vi "get_stage_info.vi"(8 "error in (no error)":errorcluster, 10 "repo_type":string, 11 "node in":refnum<k20>) -> (0 "error out":errorcluster, 2 "Stage info":T1(array[cluster]), 3 "node out":refnum<k20>)   [LabVIEW 2010, in "XML_repo_library.lvlib"]
uses:
  XML_repo_library.lvlib
  <vilib>/xml/Close Reference(Node).vi
  <vilib>/xml/NI_XML.lvlib
  C:/Program Files (x86)/National Instruments/LabVIEW 2010/resource/objmgr/DOMUserDefRef.rc
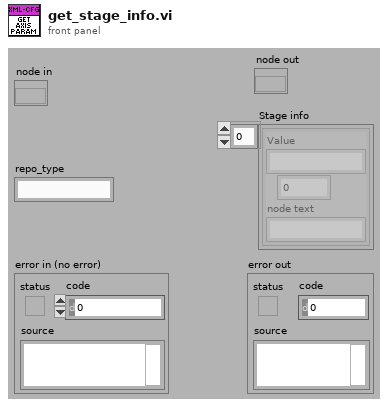
[diagram p1: front panel]
types:
  T1 = cluster{"Value":string, i32, "node text":string}[]
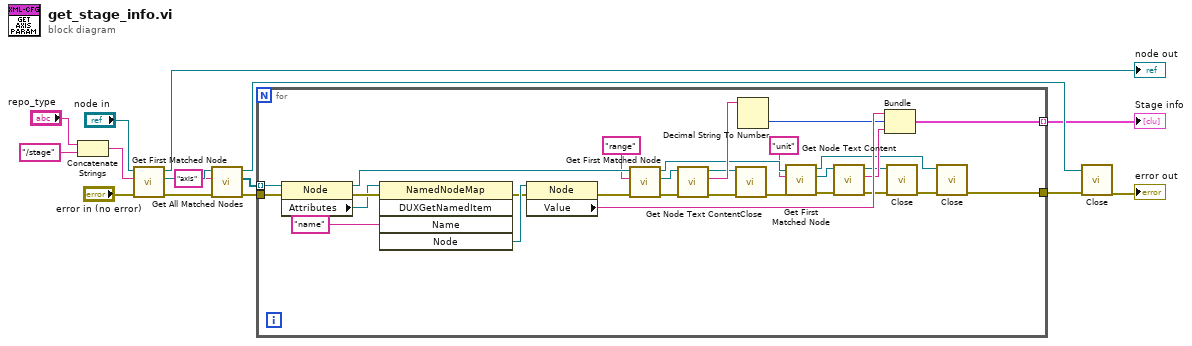
[diagram p0: block diagram]
diagram:
  n1 = Concatenate Strings("repo_type", "/stage" ("param_name")) -> (w15:string)
  n2 = call <vilib>:"Get First Matched Node.vi"("error in (no error)"="error in (no error)", "XPath expression"=w15, "node in"="node in") -> ("error out"=w9:errorcluster, "node result"=w10:refnum<k20>, "node out"=→"node out":refnum<k20>)  [unwired: 6 in]
  n3 = call <vilib>:"Get All Matched Nodes.vi"("error in (no error)"=w9, "XPath expression"="axis", "node in"=w10) -> ("error out"=w7:errorcluster, "node result array"=w8:refnum<k20>[], "node out"=w5:refnum<k20>)  [unwired: 6 in]
  n4 = for {
    tunnel: w8 -> [w38] mode=indexing
    tunnel: w7 -> [w39]
    tunnel: [w17] -> w6
    tunnel: [w16] -> w3 mode=indexing
    n5 = property class="Node"(reference=w38, error in=w39) -> (reference out=w36:refnum<k20>, error out=w44:errorcluster, "Attributes"=w43:refnum<k20>)
    n6 = invoke class="NamedNodeMap" method="DUXGetNamedItem"(reference=w43, error in=w44, "Name"="name") -> (error out=w40:errorcluster, "Node"=w41:refnum<k20>)  [unwired: 2 in, 3 out]
    n7 = property class="Node"(reference=w41, error in=w40) -> (error out=w37:errorcluster, "Value"=w26:string)  [unwired: 1 out]
    n8 = call <vilib>:"Get First Matched Node.vi"("error in (no error)"=w37, "XPath expression"="range", "node in"=w36) -> ("error out"=w34:errorcluster, "node result"=w33:refnum<k20>, "node out"=w28:refnum<k20>)  [unwired: 6 in]
    n9 = call <vilib>:"Get Node Text Content.vi"("error in (no error)"=w34, "node in"=w33) -> ("error out"=w30:errorcluster, "node text"=w32:string, "node out"=w31:refnum<k20>)  [unwired: 7 in]
    n10 = call-poly <vilib>:"Close.vi"("error in (no error)"=w30, "node"=w31) -> ("error out"=w29:errorcluster)  [unwired: 7 in]
    n11 = Decimal String To Number(string=w32) -> (number=w25:i32)  [unwired: 2 in, 1 out]
    n12 = call <vilib>:"Get First Matched Node.vi"("error in (no error)"=w29, "XPath expression"="unit", "node in"=w28) -> ("error out"=w24:errorcluster, "node result"=w23:refnum<k20>, "node out"=w18:refnum<k20>)  [unwired: 6 in]
    n13 = call <vilib>:"Get Node Text Content.vi"("error in (no error)"=w24, "node in"=w23) -> ("error out"=w21:errorcluster, "node text"=w22:string, "node out"=w20:refnum<k20>)  [unwired: 7 in]
    n14 = Bundle("Value"=w26, w25, "node text"=w22) -> (w16:cluster{"Value":string, i32, "node text":string})  [unwired: 1 in]
    n15 = call-poly <vilib>:"Close.vi"("error in (no error)"=w21, "node"=w20) -> ("error out"=w19:errorcluster)  [unwired: 7 in]
    n16 = call-poly <vilib>:"Close.vi"("error in (no error)"=w19, "node"=w18) -> ("error out"=w17:errorcluster)  [unwired: 7 in]
  }
  "Stage info" <- w3
  n17 = call-poly <vilib>:"Close.vi"("error in (no error)"=w6, "node"=w5) -> ("error out"=→"error out":errorcluster)  [unwired: 7 in]
